vi "DBInsertToTable-Log.vi"(8 "error in (no error)":errorcluster, 9 "message value":variant, 11 "ProcessState in":T1) -> (0 "error out":errorcluster, 3 "ProcessState out":T1)   [LabVIEW 2015, in "FileHandler.lvlib"]
uses:
  FileHandler.lvlib
  controls/ProcessState.ctl
  <vilib>/drjdpowell/SQLite Library/SQL Connection/Connection.lvclass
  controls/Record.ctl
  <vilib>/drjdpowell/SQLite Library/SQL Statement/SQL Statement.lvclass/SQL Statement.ctl
  <vilib>/drjdpowell/SQLite Library/SQL Statement/Bind Timestamp (Text).vi
  <vilib>/drjdpowell/SQLite Library/SQL Statement/Bind Path.vi
  <vilib>/drjdpowell/SQLite Library/SQL Statement/Bind Integer.vi
  <vilib>/drjdpowell/SQLite Library/SQL Statement/Bind Text.vi
  <vilib>/drjdpowell/SQLite Library/SQL Statement/Bind Null.vi
  <vilib>/drjdpowell/SQLite Library/SQL Statement/Error Message.vi
  <vilib>/AdvancedString/Path To Command Line String.vi
  <vilib>/drjdpowell/SQLite Library/SQL Statement/SQL Statement.lvclass
  DBToolkit/DBToolkit.lvlib
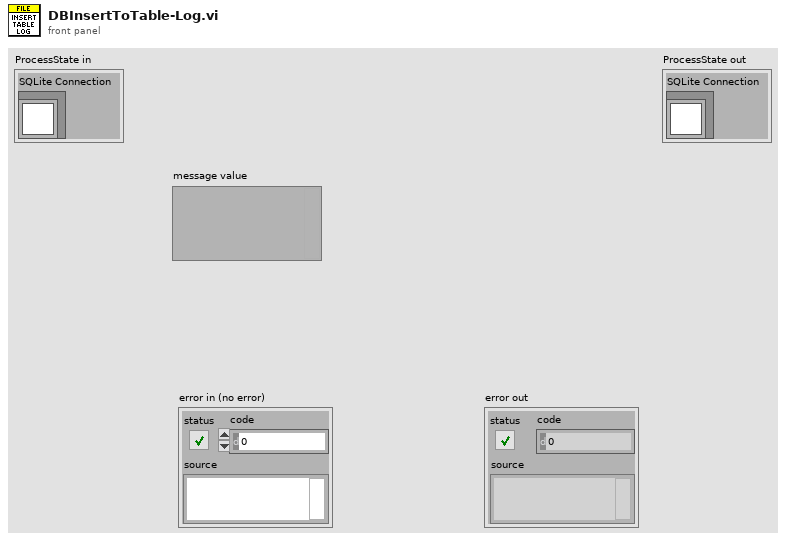
[diagram p1: front panel]
types:
  T1 = typedef "FileHandler.lvlib/ProcessState.ctl" = cluster{"SQLite Connection":refnum<class "Connection.lvclass">}
  T2 = typedef "FileHandler.lvlib/Record.ctl" = cluster{"Time":timestamp, "Path":path}
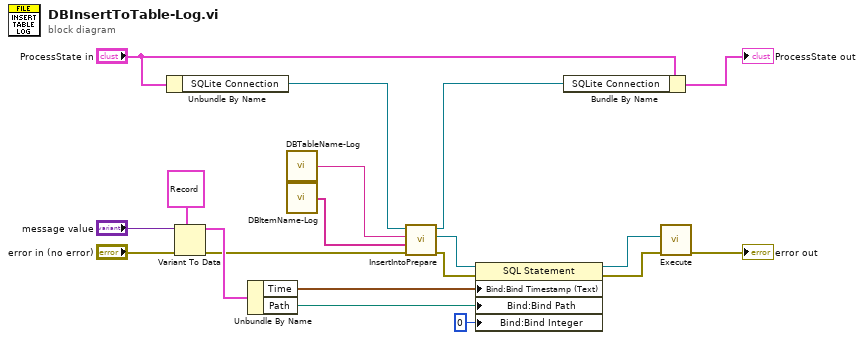
[diagram p0: block diagram]
diagram:
  n1 = Unbundle By Name("ProcessState in") -> ("SQLite Connection"=w12:refnum<class "Connection.lvclass">)
  n2 = Variant To Data(error in="error in (no error)", type=T2 {"Time"=timestamp(0 s since 1904-01-01), "Path"=path ""} ("Record"), Variant="message value") -> (data=w14:T2, error out=w13:errorcluster)
  n3 = Unbundle By Name(w14) -> ("Time"=w3:timestamp, "Path"=w2:path)
  n4 = call "DBTableName-Log.vi"() -> ("DB Table Name"=w11:string)  [unwired: 5 in]
  n5 = call "DBItemName-Log.vi"() -> ("Items"=w10:string[])  [unwired: 5 in]
  n6 = call "InsertIntoPrepare.vi"("error in (no error)"=w13, "Items"=w10, "Table Name"=w11, "SQLite Connection in"=w12) -> ("error out"=w9:errorcluster, "SQL Statement out"=w8:refnum<class "SQL Statement.lvclass">, "SQLite Connection out"=w4:refnum<class "Connection.lvclass">)  [unwired: 5 in]
  n7 = property class="SQL Statement"(reference=w8, error in=w9, "Bind:Bind Timestamp (Text)"=w3, "Bind:Bind Path"=w2, "Bind:Bind Integer"=i64 0 ("Bind:Integer")) -> (reference out=w7:refnum<class "SQL Statement.lvclass">, error out=w6:errorcluster)
  n8 = Bundle By Name(cluster="ProcessState in", "SQLite Connection"=w4) -> (→"ProcessState out":T1)
  n9 = call "Execute.vi"("error in (no error)"=w6, "SQL Statement in"=w7) -> ("error out"=→"error out":errorcluster)  [unwired: 9 in]
